vi "Set Initialization Data - Listener.vi"(8 "error in":errorcluster, 11 "Server Client in":refnum<class "Server Client.lvclass">) -> (0 "error out":errorcluster, 3 "Server Client out":refnum<class "Server Client.lvclass">)   [LabVIEW 2020, in "Server Client.lvclass"]
doc: "Sets the initialization data of a statically linked subWorker."
uses:
  Server Client.lvclass
  C:/Program Files (x86)/National Instruments/LabVIEW 2020/vi.lib/addons/_Workers/Library/Classes/Worker/Worker.lvclass
  Listener/Initialization Data.ctl
  Server Client.lvclass/Server Client.ctl
  Listener/Listener.lvclass
  <vilib>/addons/_Workers/Library/Classes/Worker/Worker.lvclass
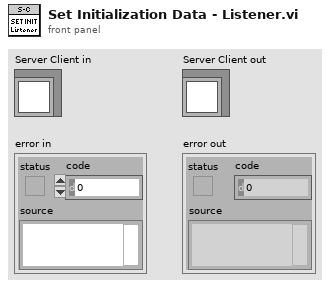
[diagram p1: front panel]
types:
  T1 = typedef "Listener.lvclass/Initialization Data.ctl" = cluster{"String":string, "port":u16}
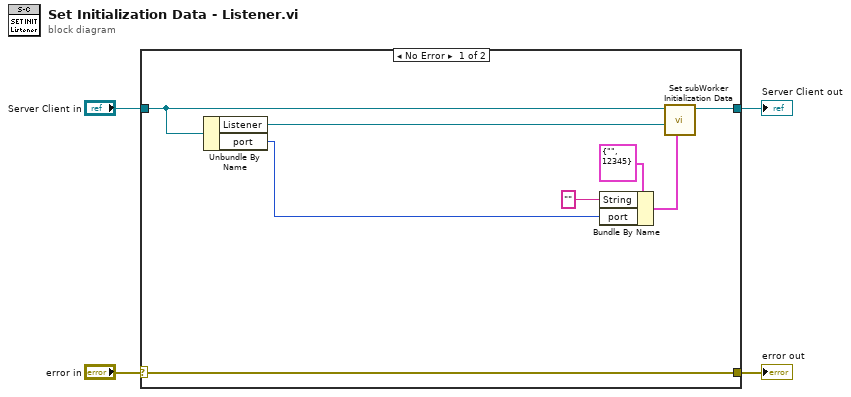
[diagram p0: block diagram]
diagram:
  n1 = case shown="No Error" "error in" {
    selector: "error in" -> [w12 w14]
    tunnel: [w12 w14] -> w3
    tunnel: [w10 w13] -> w2
    tunnel: "Server Client in" -> [w9 w13]
    frame No Error {
      n2 = Unbundle By Name(w9) -> ("Listener"=w11:refnum<class "Listener.lvclass">, "port"=w5:u16)
      n3 = Bundle By Name(cluster=T1 {"String"="", "port"=12345} ("Initialization Data"), "String"="" ("Placeholder"), "port"=w5) -> (w7:T1)
      n4 = call <vilib>:"Set subWorker Initialization Data.vi"("Initialization Data"=w7, "subWorker"=w11, "Worker"=w9) -> ("Worker out"=w10:refnum<class "Server Client.lvclass">)  [unwired: 8 in]
    }
    frame Error {
    }
  }
  "error out" <- w3
  "Server Client out" <- w2
